vi "append source thread and state to error.vi"(8 "error in (no error)":errorcluster, 11 "String":string) -> (0 "error out":errorcluster)   [LabVIEW 2012]
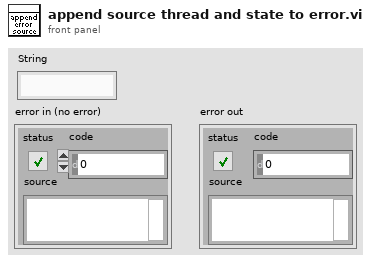
[diagram p1: front panel]
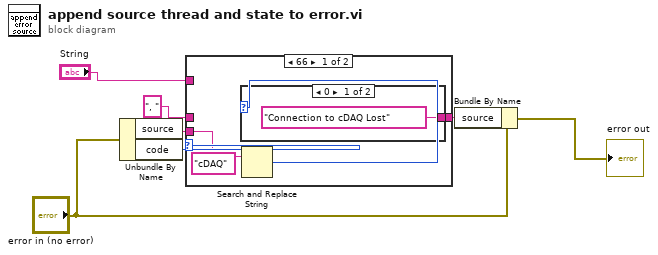
[diagram p0: block diagram]
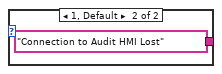
[diagram p2: hidden frame]
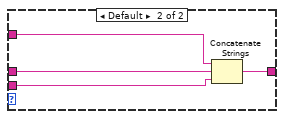
[diagram p3: hidden frame]
diagram:
  n1 = Unbundle By Name("error in (no error)") -> ("source"=w4:string, "code"=w1:i32)
  n2 = case shown="66" w1 {
    tunnel: ", " ("string") -> [_ w17]
    tunnel: "String" -> [_ w16]
    tunnel: [w11 w15] -> w5
    tunnel: w4 -> [w10 w14]
    frame 66 {
      n3 = Search and Replace String(input string=w10, search string="cDAQ") -> (number of replacements=w8:i32)  [unwired: 6 in, 3 out]
      n4 = case shown="0" w8 {
        tunnel: ["Connection to cDAQ Lost" "Connection to Audit HMI Lost"] -> w11
        frame 0 {
        }
        frame 1, Default {
        }
      }
    }
    frame Default {
      n5 = Concatenate Strings(w16, w17, w14) -> (w15:string)
    }
  }
  n6 = Bundle By Name(cluster="error in (no error)", "source"=w5) -> (→"error out":errorcluster)
